vi "ViHandler.Initialize.vi"(8 "Error In":errorcluster) -> (0 "Error out":errorcluster, 3 "ViHandler":refnum<data-value>)   [LabVIEW 2016, in "ViHandler.lvclass"]
uses:
  ViHandler.lvclass
  ObjectHandler/ObjectHandler.GetObjectWType.ctl
  ObjectHandler/ObjectHandler.ObjectType.ctl
  ObjectHandler/ObjectHandler.ObjectMessage.ctl
  ObjectHandler/ObjectHandler.ObjectWType.ctl
  ObjectHandler/ObjectHandler.lvclass
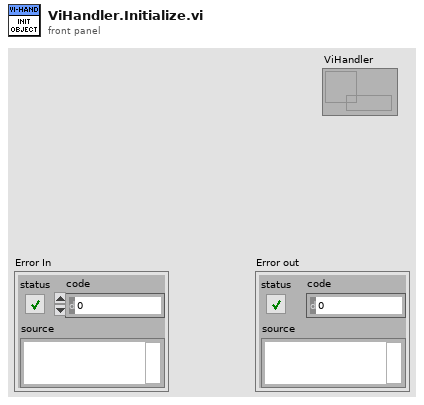
[diagram p1: front panel]
types:
  T1 = typedef "ObjectHandler.lvclass/ObjectHandler.ObjectMessage.ctl" = cluster{"Name":string, "ObjectWType":T2}
  T2 = typedef "ObjectHandler.lvclass/ObjectHandler.ObjectWType.ctl" = cluster{"ObjectType":T3, "Object":variant}
  T3 = typedef "ObjectHandler.lvclass/ObjectHandler.ObjectType.ctl" = enum16{"undefined", "ObjectHandler", "ViHandler", "ErrorHandler", "CentralStorage", "Hausmodell", "Sondenmodell", "Wärmepumpe", "Umgebung"}
  T4 = typedef "ObjectHandler.lvclass/ObjectHandler.GetObjectWType.ctl" = cluster{"Name":string, "Caller":string}
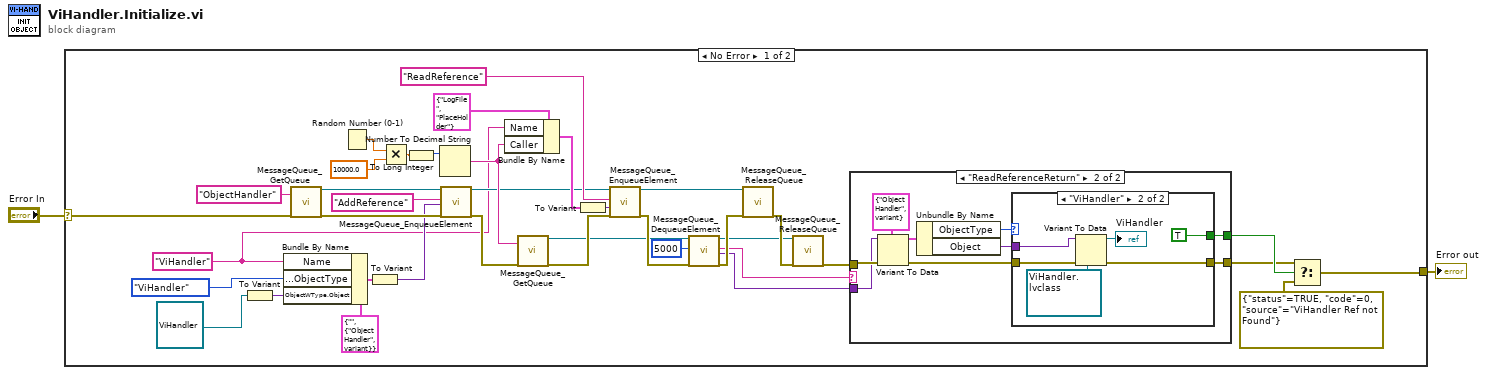
[diagram p0: block diagram]
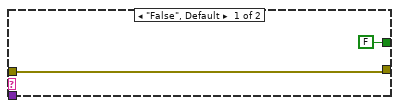
[diagram p2: hidden frame]
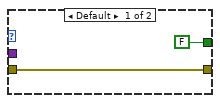
[diagram p3: hidden frame]
diagram:
  n1 = case shown="No Error" "Error In" {
    selector: "Error In" -> [w5 w60]
    tunnel: [w40 w60] -> w2
    frame No Error {
      w4 = "ViHandler" ("Name")
      n2 = To Variant(anything=refnum<class "ViHandler.lvclass"> refnum ("ViHandler.lvclass")) -> (Variant=w12:variant)
      n3 = Bundle By Name(cluster=T1 {"Name"="", "ObjectWType"={"ObjectType"=enum."ObjectHandler", "Object"=variant(refnum<data-value> refnum)}} ("ObjectMessage"), "Name"=w4, "ObjectWType.ObjectType"=ObjectHandler.ObjectType."ViHandler" ("ObjectType"), "ObjectWType.Object"=w12) -> (w11:T1)
      n4 = call "MessageQueue_GetQueue.vi"("Name"="ObjectHandler", "ErrorIn"=w5) -> ("QueueOut"=w14:refnum<queue>, "ErrorOut"=w15:errorcluster)  [unwired: 15 in, 1 out]
      n5 = Random Number (0-1)() -> (number: 0 to 1=w39:dbl)
      n6 = To Variant(anything=w11) -> (Variant=w10:variant)
      n7 = Multiply(x=w39, y=10000.0) -> (x*y=w37:dbl)
      n8 = To Long Integer(number=w37) -> (32bit integer=w36:i32)
      n9 = Number To Decimal String(number=w36) -> (decimal integer string=w21:string)  [unwired: 1 in]
      n10 = call "MessageQueue_EnqueueElement.vi"("QueueIn"=w14, "Message"="AddReference", "Data"=w10, "ErrorIn"=w15) -> ("QueueOut"=w6:refnum<queue>, "ErrorOut"=w7:errorcluster)  [unwired: 14 in]
      n11 = Bundle By Name(cluster=T4 {"Name"="LogFile", "Caller"="PlaceHolder"} ("GetRefInput"), "Name"=w4, "Caller"=w21) -> (w20:T4)
      n12 = call "MessageQueue_GetQueue.vi"("Name"=w21, "ErrorIn"=w7) -> ("QueueOut"=w30:refnum<queue>, "ErrorOut"=w35:errorcluster)  [unwired: 15 in, 1 out]
      n13 = To Variant(anything=w20) -> (Variant=w25:variant)
      n14 = call "MessageQueue_EnqueueElement.vi"("QueueIn"=w6, "Message"="ReadReference", "Data"=w25, "ErrorIn"=w35) -> ("QueueOut"=w31:refnum<queue>, "ErrorOut"=w34:errorcluster)  [unwired: 14 in]
      n15 = call "MessageQueue_DequeueElement.vi"("QueueIn"=w30, "Timeout"=5000, "ErrorIn"=w34) -> ("QueueOut"=w29:refnum<queue>, "Message"=w27:string, "Data"=w23:variant, "ErrorOut"=w33:errorcluster)  [unwired: 12 in, 1 out]
      n16 = call "MessageQueue_ReleaseQueue.vi"("QueueIn"=w31, "ErrorIn"=w33) -> ("ErrorOut"=w32:errorcluster)  [unwired: 15 in, 2 out]
      n17 = call "MessageQueue_ReleaseQueue.vi"("QueueIn"=w29, "ErrorIn"=w32) -> ("ErrorOut"=w24:errorcluster)  [unwired: 15 in, 2 out]
      n18 = case shown="\"ReadReferenceReturn\"" w27 {
        tunnel: w24 -> [w41 w51]
        tunnel: w23 -> [_ w50]
        tunnel: [w41 w44] -> w18
        tunnel: [FALSE w43] -> w19
        frame "False", Default {
        }
        frame "ReadReferenceReturn" {
          n19 = Variant To Data(error in=w51, type=T2 {"ObjectType"=enum."ObjectHandler", "Object"=variant} ("ObjectWType"), Variant=w50) -> (data=w48:T2, error out=w45:errorcluster)
          n20 = Unbundle By Name(w48) -> ("ObjectType"=w47:T3, "Object"=w46:variant)
          n21 = case shown="\"ViHandler\"" w47 {
            tunnel: w46 -> [_ w59]
            tunnel: w45 -> [w53 w58]
            tunnel: [w53 w57] -> w44
            tunnel: [FALSE TRUE] -> w43
            frame Default {
            }
            frame "ViHandler" {
              n22 = Variant To Data(error in=w58, type=refnum<data-value> refnum ("data value reference"), Variant=w59) -> (data=→"ViHandler":refnum<data-value>, error out=w57:errorcluster)
            }
          }
        }
      }
      n23 = Select(t=w18, s=w19, f=errorcluster {"status"=TRUE, "code"=0, "source"="ViHandler Ref not Found"}) -> (s? t:f=w40:errorcluster)
    }
    frame Error {
    }
  }
  "Error out" <- w2
